vi "writeCtlsToFile.vi"(9 "ControlsToSave":refnum<vi>[](array[refnum]), 10 "path":path) -> (0 "error out":errorcluster, 3 "nameUsed":string caption="default name")   [LabVIEW 2015]
uses:
  <vilib>/NI/GXML/GXML.lvlib
panel:
  in  "FILE_NAME":string
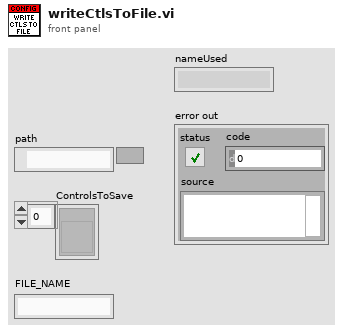
[diagram p1: front panel]
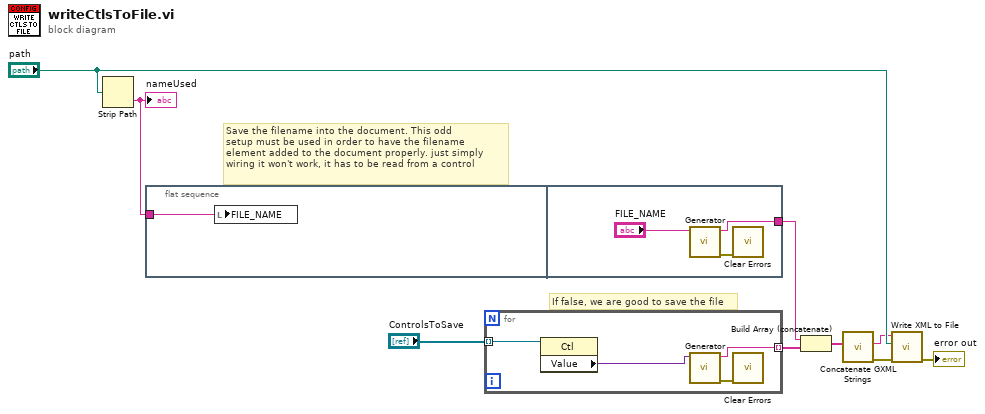
[diagram p0: block diagram]
diagram:
  # "If false, we are good to save the file"
  # "Save the filename into the document. This odd\nsetup must be used in order to have the filename\nelement added to the document properly. just simply\nwiring it won't work, it has to be read from a control"
  n1 = Strip Path(path="path") -> (name=w8:string)  [unwired: 1 out]
  "nameUsed" <- w8
  n2 = flat-sequence {
    tunnel: w8 -> [w10]
    tunnel: [w12] -> w2
    frame #0 {
      n3 = local write "FILE_NAME"(w10) -> ()
    }
    frame #1 {
      n4 = call <vilib>:"Generator.vi"("Variant"="FILE_NAME") -> ("error out"=w11:errorcluster, "XML String Out"=w12:string)  [unwired: 9 in]
      n5 = call <vilib>:"Clear Errors.vi"("error in (no error)"=w11) -> ()  [unwired: 5 in, 2 out]
    }
  }
  n6 = for {
    tunnel: "ControlsToSave" -> [w17] mode=indexing
    tunnel: [w15] -> w3 mode=indexing
    n7 = property class="Ctl"(reference=w17) -> ("Value"=w16:variant)  [unwired: 1 in, 2 out]
    n8 = call <vilib>:"Generator.vi"("Variant"=w16) -> ("error out"=w14:errorcluster, "XML String Out"=w15:string)  [unwired: 9 in]
    n9 = call <vilib>:"Clear Errors.vi"("error in (no error)"=w14) -> ()  [unwired: 5 in, 2 out]
  }
  n10 = Build Array (concatenate)(w2, w3) -> (w4:string[])
  n11 = call <vilib>:"Concatenate GXML Strings.vi"("GXML Strings"=w4) -> ("error out"=w6:errorcluster, "Concatenated GXML String"=w5:string)  [unwired: 9 in]
  n12 = call <vilib>:"Write XML to File.vi"("error in"=w6, "XML File Path"="path", "XML Input"=w5) -> ("error out"=→"error out":errorcluster)  [unwired: 8 in]
